vi "max_min.vi"(2 "b":dbl, 3 "a":dbl) -> (0 "min":dbl, 1 "max":dbl)   [LabVIEW 2017]
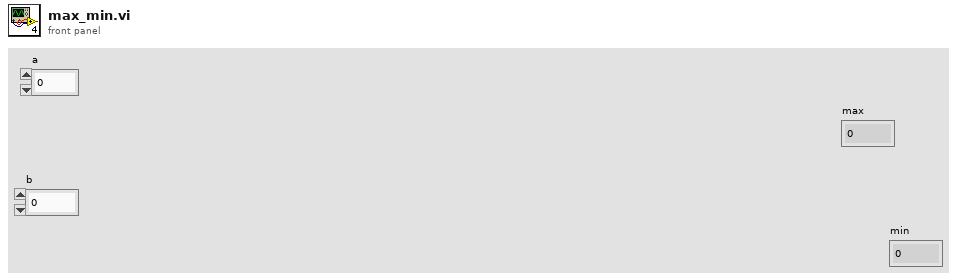
[diagram p1: front panel]
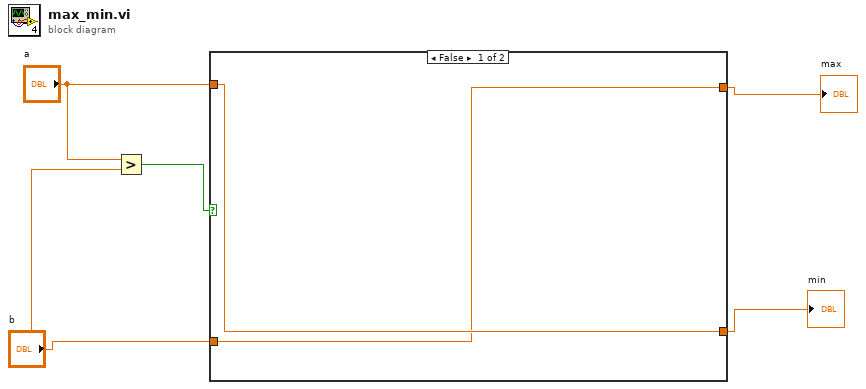
[diagram p0: block diagram]
diagram:
  n1 = Greater?(x="a", y="b") -> (0:w5:bool)
  n2 = case shown="False" w5 {
    tunnel: "a" -> [w7 w9]
    tunnel: [w6 w9] -> w3
    tunnel: "b" -> [w6 w8]
    tunnel: [w7 w8] -> w1
    frame False {
    }
    frame True {
    }
  }
  "max" <- w3
  "min" <- w1
